vi "Generation of Triangular waves from sine waves.vi"() -> ()   [LabVIEW 2009]
uses:
  <vilib>/Analysis/NI_AALBase.lvlib
panel:
  out "Individual sine waves":dbl[][](graph)
  in  "stop":bool
  in  "# of Sines":i32(slide) step=1 scale=0.0..50.0
  out "Waveform Graph":dbl[](graph)
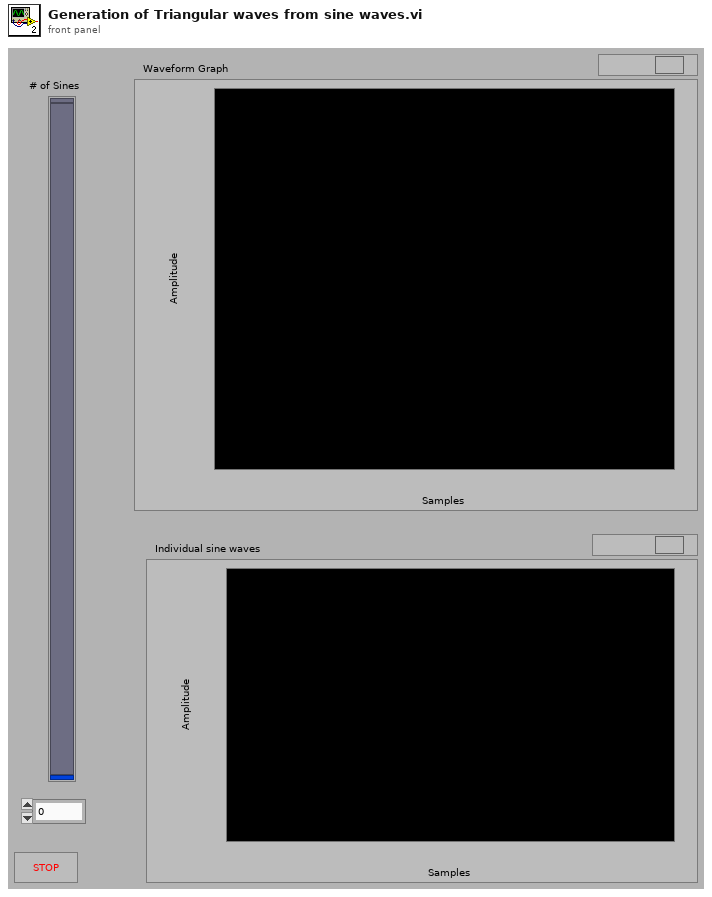
[diagram p1: front panel]
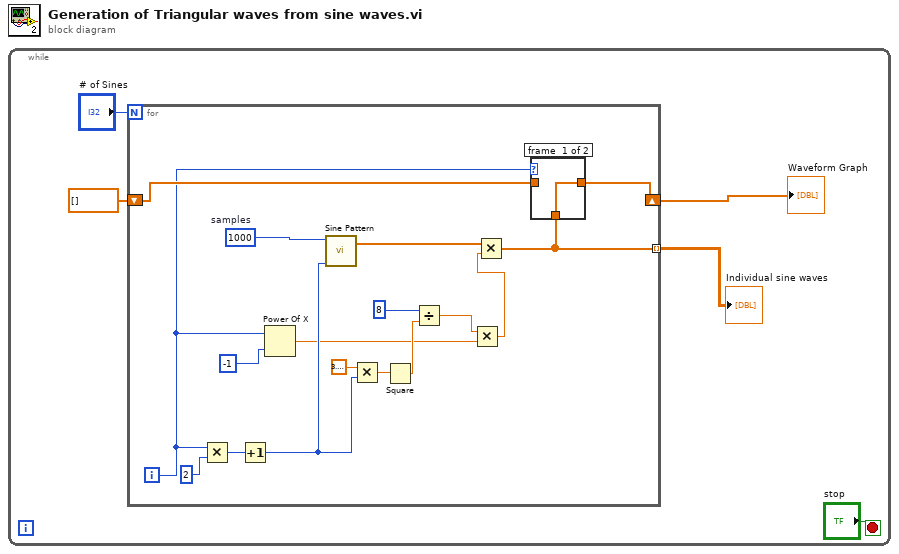
[diagram p0: block diagram]
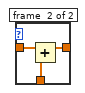
[diagram p2: hidden frame]
diagram:
  n1 = while {
    stop <- "stop" stop-if-true
    n2 = for {
      N: "# of Sines" -> [_]
      shift-right: [w19] -> w5
      shift-left: dbl[] [] ("Sinusoidal Pattern") -> [w20]
      tunnel: [w9] -> w1 mode=indexing
      i -> [w10]
      w22 = 1000  # samples
      n3 = Multiply(x=w10, y=2) -> (x*y=w17:i32)
      n4 = Increment(x=w17) -> (x+1=w14:i32)
      n5 = Power Of X(1:-1, 2:w10) -> (0:w6:dbl)
      n6 = call <vilib>:"Sine Pattern.vi"("cycles"=w14, "samples"=w22) -> ("Sinusoidal Pattern"=w21:dbl[])  [unwired: 2 in, 1 out]
      n7 = Multiply(x=3.141592653589793, y=w14) -> (x*y=w13:dbl)
      n8 = Square(x=w13) -> (x^2=w12:dbl)
      n9 = Divide(x=8 ("y"), y=w12) -> (x/y=w8:dbl)
      n10 = Multiply(x=w8, y=w6) -> (x*y=w7:dbl)
      n11 = Multiply(x=w21, y=w7) -> (x*y=w9:dbl[])
      n12 = case shown="Default" w10 {
        tunnel: [w23 w26] -> w19
        tunnel: w20 -> [_ w25]
        tunnel: w9 -> [w23 w24]
        frame #0 {
        }
        frame #1 {
          n13 = Add(x=w25, y=w24) -> (x+y=w26:dbl[])
        }
      }
    }
    "Waveform Graph" <- w5
    "Individual sine waves" <- w1
  }
